vi "write_command.vi"(7 "read (T)":bool=TRUE, 8 "error in (no error)":errorcluster, 10 "string to write":string, 11 "StageMH110930Scientifica in":refnum<class "StageMMS2015ASIfromScientifica.lvclass">) -> (0 "error out":errorcluster, 2 "read string":string, 3 "StageMH110930Scientifica out":refnum<class "StageMMS2015ASIfromScientifica.lvclass">, 4 "approved response?":bool)   [LabVIEW 2010, in "StageMMS2015ASIfromScientifica.lvclass"]
uses:
  StageMMS2015ASIfromScientifica.lvclass
  common/classes/ErrorController/ErrorController/class_data.vi
  common/classes/ErrorController/ErrorController/ErrorController.lvclass
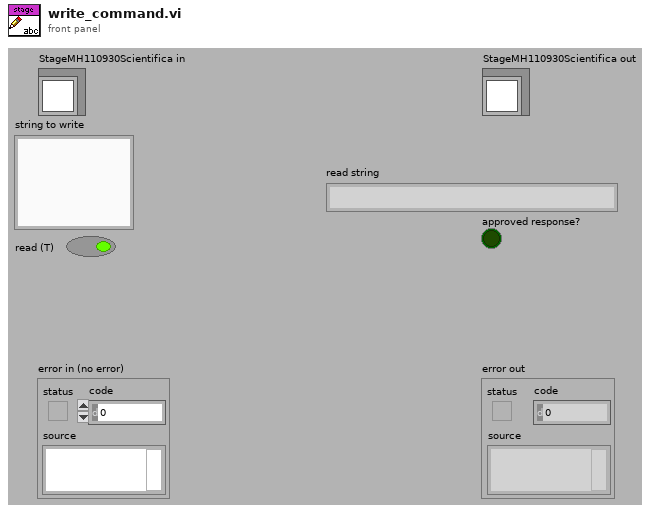
[diagram p1: front panel]
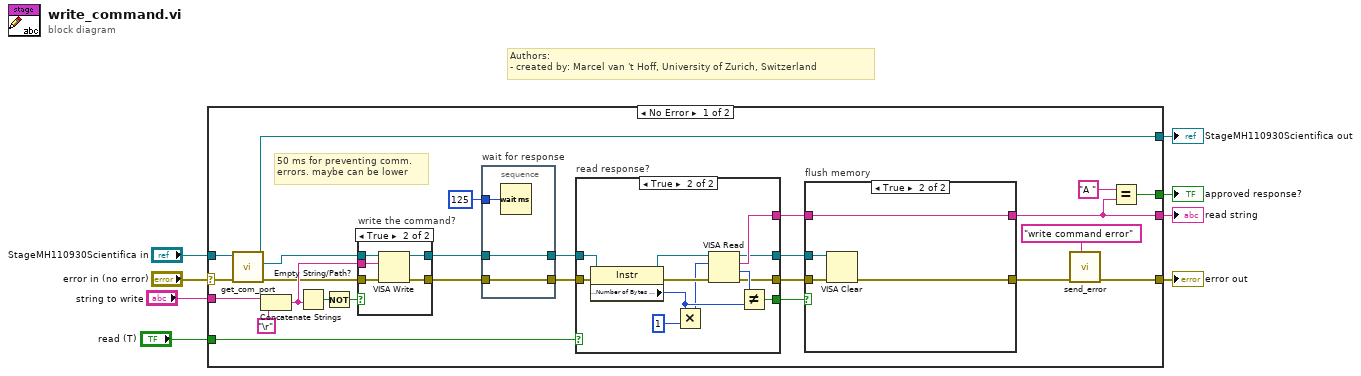
[diagram p0: block diagram]
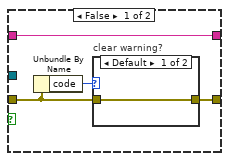
[diagram p2: hidden frame]
diagram:
  # "Authors: \n- created by: Marcel van 't Hoff, University of Zurich, Switzerland"
  n1 = case shown="No Error" "error in (no error)" {
    selector: "error in (no error)" -> [w32 w69]
    tunnel: [w14 w69] -> w7
    tunnel: [w33 w68] -> w5
    tunnel: "StageMH110930Scientifica in" -> [w34 w68]
    tunnel: "string to write" -> [w30 _]
    tunnel: "read (T)" -> [w19 _]
    tunnel: [w12 _] -> w2
    tunnel: [w10 _] -> w1
    frame No Error {
      # "50 ms for preventing comm.\nerrors. maybe can be lower"
      n2 = call-dynamic "get_com_port.vi"("error in (no error)"=w32, "StageMH110930Scientifica in"=w34) -> ("error out"=w25:errorcluster, "serial port name"=w28:refnum<visa-resource-name>, "StageMH110930Scientifica out"=w33:refnum<class "StageMMS2015ASIfromScientifica.lvclass">)  [unwired: 7 in]
      n3 = Concatenate Strings(w30, "\r") -> (w26:string)
      n4 = Empty String/Path?(string/path=w26) -> (empty?=w29:bool)
      n5 = Not(x=w29) -> (.not. x?=w27:bool)
      n6 = case "write the command?" shown="True" w27 {
        tunnel: [w62 w67] -> w23
        tunnel: w28 -> [w61 w66]
        tunnel: w25 -> [w62 w65]
        tunnel: [w61 w64] -> w24
        tunnel: w26 -> [_ w63]
        frame False {
        }
        frame True {
          n7 = VISA Write(VISA resource name=w66, write buffer=w63, error in (no error)=w65) -> (VISA resource name out=w64:refnum<visa-resource-name>, error out=w67:errorcluster)  [unwired: 1 out]
        }
      }
      n8 = stacked-sequence "wait for response" {
        tunnel: w23 -> [w60]
        tunnel: [w60] -> w20
        tunnel: w24 -> [w59]
        tunnel: [w59] -> w21
        tunnel: u32 125 ("delay before read (ms)") -> [w58]
        frame #0 {
          n9 = Wait (ms)(milliseconds to wait=w58) -> ()  [unwired: 1 out]
        }
      }
      n10 = case "read response?" shown="True" w19 {
        tunnel: w20 -> [w45 w55]
        tunnel: [w45 w49] -> w16
        tunnel: w21 -> [w44 w57]
        tunnel: [_ w53] -> w17
        tunnel: [_ w51] -> w9
        tunnel: [w44 w50] -> w18
        frame False {
        }
        frame True {
          n11 = property class="Instr"(reference=w57, error in=w55) -> (reference out=w56:refnum<visa-resource-name>, error out=w54:errorcluster, "Serial Settings:Number of Bytes at Serial Port"=w48:u32)
          n12 = Multiply(x=w48, y=u32 1) -> (x*y=w46:u32)
          n13 = VISA Read(VISA resource name=w56, byte count=w46, error in (no error)=w54) -> (VISA resource name out=w50:refnum<visa-resource-name>, read buffer=w53:string, return count=w52:u32, error out=w49:errorcluster)
          n14 = Not Equal?(x=w52, y=w48) -> (x != y?=w51:bool)
        }
      }
      n15 = case "flush memory" shown="True" w9 {
        tunnel: w16 -> [w36 w43]
        tunnel: w18 -> [_ w42]
        tunnel: [w38 w41] -> w12
        tunnel: w17 -> [w38 w41]
        tunnel: [w35 w40] -> w15
        frame False {
          n16 = Unbundle By Name(w36) -> ("code"=w37:i32)
          n17 = case "clear warning?" shown="Default" w37 {
            tunnel: w36 -> [w39 _]
            tunnel: [w39 _] -> w35
            frame Default {
            }
            frame 1073676294 {
            }
          }
        }
        frame True {
          n18 = VISA Clear(VISA resource name=w42, error in (no error)=w43) -> (error out=w40:errorcluster)  [unwired: 1 out]
        }
      }
      n19 = call "send_error.vi"("additional message"="write command error", "error in (no error)"=w15) -> ("error out"=w14:errorcluster)  [unwired: 9 in]
      n20 = Equal?(x="A " ("y"), y=w12) -> (x = y?=w10:bool)
    }
    frame Error {
    }
  }
  "error out" <- w7
  "StageMH110930Scientifica out" <- w5
  "read string" <- w2
  "approved response?" <- w1
